vi "Pre Launch Init.vi"(11 "ObservingModel In":refnum<class "ObservingModel.lvclass">) -> (0 "error out":errorcluster, 3 "ObservingModel Out":refnum<class "ObservingModel.lvclass">)   [LabVIEW 2017, in "TestPubSubRouting.lvlib" / "ObservingModel.lvclass"]
doc: "(<B>Filename</B>: Actor Framework.lvlib:Actor.lvclass:Pre Launch Init.vi)\n\nDefines behavior that occurs after the Launch Nested Actor method is invoked but before the actor's Actor Core method begins running.\n\nBy default, this method does nothing. A descendant class may override it to define behavior."
uses:
  ObservingModel.lvclass
  C:/Git/mva-framework/Source/Framework/IObserver/IObserver/IObserver.lvclass
  <vilib>/ActorFramework/Actor/Actor.lvclass/Actor.ctl
  <vilib>/ActorFramework/Message Enqueuer/Message Enqueuer.lvclass/Message Enqueuer.ctl
  Source/Framework/SubscriptionPolicy/ValueChangeSubscription/ValueChangeSubscription.lvclass/ValueChangeSubscription.ctl
  Source/Framework/IMediator/SubscriptionRequest/SubscriptionRequest.lvclass/SubscriptionRequest.ctl
  Source/Framework/IObserver/IObserver Messages/Subscribe Msg/Subscribe Msg.lvclass/Subscribe Msg.ctl
  Source/Framework/IMediator/SubscriptionRequest/Pack Subscription Request.vi
  <vilib>/ActorFramework/Actor/Read Self Enqueuer.vi
  Source/Framework/SubscriptionPolicy/BasicSubscription/New Basic Subscription.vi
  Source/Framework/SubscriptionPolicy/ValueChangeSubscription/New Value Change Subscription.vi
  Source/Framework/IObserver/IObserver Messages/Subscribe Msg/Send Subscribe.vi
  <vilib>/ActorFramework/Message Enqueuer/Init from Existing Queue.vi
  <vilib>/ActorFramework/Message Enqueuer/Enqueue.vi
  Source/Framework/SubscriptionPolicy/ValueChangeSubscription/ValueChangeSubscription.lvclass
  C:/Git/mva-framework/Source/Framework/IMediator/ISubscriptionPolicy/ISubscriptionPolicy.lvclass
  Source/Framework/IObserver/IObserver/IObserver.lvclass
  C:/Program Files (x86)/National Instruments/LabVIEW 2017/vi.lib/ActorFramework/Actor/Actor.lvclass
  Source/Framework/IObserver/ActorDataBinding/ActorDataBinding.lvclass
  C:/Git/mva-framework/gpm_packages/@cs/transport/Source/ITransport/ITransport.lvclass
  Source/Framework/IObserver/IObserver Messages/Subscribe Msg/Subscribe Msg.lvclass
  C:/Program Files (x86)/National Instruments/LabVIEW 2017/vi.lib/ActorFramework/Message/Message.lvclass
  <vilib>/ActorFramework/Message Priority Queue/Priority Enqueue.vi
  Source/Framework/IMediator/ISubscriptionPolicy/Open Subscription Policy.vi
  Source/Framework/IObserver/ActorDataBinding/New Actor Data Binding Transport.vi
  Source/Framework/IModel/IModel/IModel.lvclass
  Source/Framework/IMediator/SubscriptionRequest/SubscriptionRequest.lvclass
  <vilib>/ActorFramework/Message Enqueuer/Message Enqueuer.lvclass
  Source/Framework/SubscriptionPolicy/BasicSubscription/BasicSubscription.lvclass
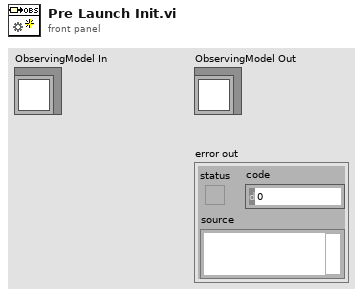
[diagram p1: front panel]
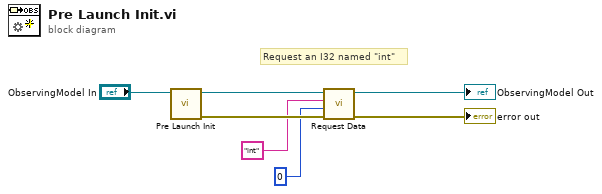
[diagram p0: block diagram]
diagram:
  # "Request an I32 named \"int\""
  n1 = call-parent "Pre Launch Init.vi"("IModel in"="ObservingModel In") -> ("error out"=w4:errorcluster, "IModel out"=w7:refnum<class "ObservingModel.lvclass">)  [unwired: 9 in]
  n2 = call "Request Data.vi"("error in (no error)"=w4, "Data Type"=0, "Datum Name"="int", "IObserver in"=w7) -> ("error out"=→"error out":errorcluster, "IObserver out"=→"ObservingModel Out":refnum<class "ObservingModel.lvclass">)  [unwired: 5 in, 1 out]
